vi "tb_ Four 64 bit to 256 bit pack.vi"() -> (3 "Pass?":bool)   [LabVIEW 2011]
uses:
  DRAM/2 Bank DRAM/Data Type (256).ctl
panel:
  out "Collected Data":T1[](array[typedef])
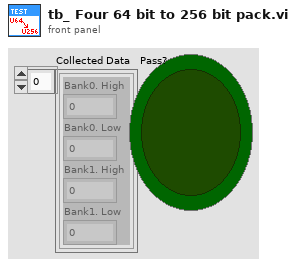
[diagram p1: front panel]
types:
  T1 = typedef "Data Type (256).ctl" = cluster{"Bank0. High":u64, "Bank0. Low":u64, "Bank1. High":u64, "Bank1. Low":u64}
  T2 = cluster{"First":u64, "Second":u64, "Third":u64, "Fourth":u64}
  T3 = cluster{"Bank0. High":bool, "Bank0. Low":bool, "Bank1. High":bool, "Bank1. Low":bool}
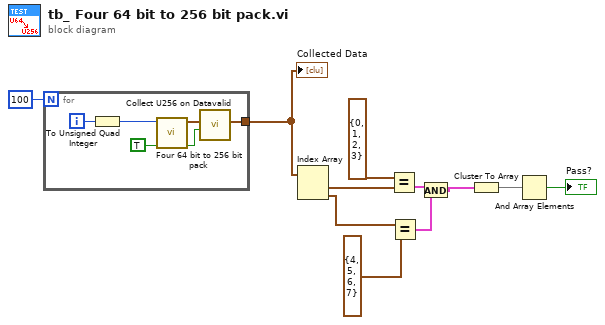
[diagram p0: block diagram]
diagram:
  n1 = for {
    N: 100 -> [_]
    tunnel: [w12] -> w10
    i -> [w17]
    n2 = To Unsigned Quad Integer(1:w17) -> (0:w16:u64)
    n3 = call "Four 64 bit to 256 bit pack.vi"("Input Valid"=TRUE, "Input Data"=w16) -> ("Output Valid"=w14:bool, "Output Data"=w13:T2)  [unwired: 8 in]
    n4 = call "Collect U256 on Datavalid.vi"("Data Valid"=w14, "Input Data"=w13) -> ("Collected Data"=w12:T1[])  [unwired: 9 in]
  }
  "Collected Data" <- w10
  n5 = Index Array(array=w10) -> (element #1=w9:T1, element #2=w8:T1)  [unwired: 2 in]
  n6 = Equal?(x=T1 {"Bank0. High"=0, "Bank0. Low"=1, "Bank1. High"=2, "Bank1. Low"=3} ("y"), y=w9) -> (x = y?=w5:T3)
  n7 = Equal?(x=w8, y=T1 {"Bank0. High"=4, "Bank0. Low"=5, "Bank1. High"=6, "Bank1. Low"=7}) -> (x = y?=w4:T3)
  n8 = And(x=w5, y=w4) -> (x .and. y?=w3:T3)
  n9 = Cluster To Array(cluster=w3) -> (array=w2:bool[])
  n10 = And Array Elements(Boolean array=w2) -> (logical AND=→"Pass?":bool)
